vi "Reset_To_Zero.vi"(8 "error in":errorcluster, 11 "X-CAN Session in":refnum<class "X-CAN.lvclass">) -> (0 "error out":errorcluster, 3 "X-CAN Session out":refnum<class "X-CAN.lvclass">)   [LabVIEW 2015]
uses:
  <vilib>/Stratom, Inc/X-CAN for myRIO (API)/X-CAN Class/X-CAN.lvclass
  <vilib>/Stratom, Inc/X-CAN for myRIO (API)/X-CAN Class/Type Definitions/CANFrame.ctl
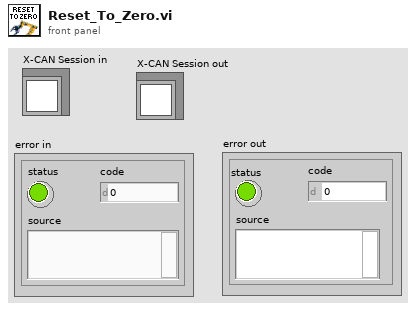
[diagram p1: front panel]
types:
  T1 = typedef "X-CAN.lvclass/CANFrame.ctl" = cluster{"identifier":u32, "extended?":bool, "echo?":bool, "payload":u8[], "timestamp":timestamp}
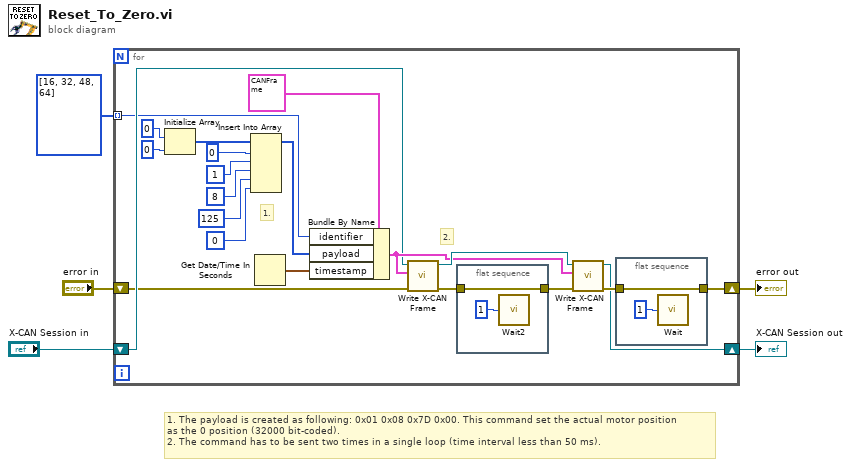
[diagram p0: block diagram]
diagram:
  # "1. The payload is created as following: 0x01 0x08 0x7D 0x00. This command set the actual motor position\nas the 0 position (32000 bit-coded).\n2. The command has to be sent two times in a single loop (time interval less than 50 ms)."
  n1 = for {
    shift-right: [w8] -> w3
    shift-left: "X-CAN Session in" -> [w10]
    shift-right: [w7] -> w2
    shift-left: "error in" -> [w9]
    tunnel: u8[] [16, 32, 48, 64] ("identifier") -> [w6] mode=indexing
    # "2."
    # "1."
    n2 = Initialize Array(u16 0 ("element"), 0 ("dimension size")) -> (w18:u16[])
    n3 = Insert Into Array(array=w18, index=0, new element #1=u8 1 ("new element/subarray"), new element #2=u8 8 ("new element/subarray"), new element #3=u8 125 ("new element/subarray"), new element #4=u8 0 ("new element/subarray")) -> (w15:u16[])
    n4 = Get Date/Time In Seconds() -> (seconds since 1Jan1904=w22:timestamp)
    n5 = Bundle By Name(cluster=T1 {"identifier"=0, "extended?"=FALSE, "echo?"=FALSE, "payload"=[], "timestamp"=timestamp(0 s since 1904-01-01)} ("CAN Frame"), "identifier"=w6, "payload"=w15, "timestamp"=w22) -> (w13:T1)
    n6 = call <vilib>:"Write X-CAN Frame.vi"("error in"=w9, "CAN Frame"=w13, "X-CAN Session in"=w10) -> ("error out"=w24:errorcluster, "X-CAN Session out"=w25:refnum<class "X-CAN.lvclass">)  [unwired: 7 in]
    n7 = flat-sequence {
      tunnel: w24 -> [w27]
      tunnel: [w27] -> w23
      frame #0 {
        n8 = call "Wait2"("Count(mSec)"=u32 1 ("milliseconds to wait")) -> ()  [unwired: 1 out]
      }
    }
    n9 = call <vilib>:"Write X-CAN Frame.vi"("error in"=w23, "CAN Frame"=w13, "X-CAN Session in"=w25) -> ("error out"=w26:errorcluster, "X-CAN Session out"=w8:refnum<class "X-CAN.lvclass">)  [unwired: 7 in]
    n10 = flat-sequence {
      tunnel: w26 -> [w29]
      tunnel: [w29] -> w7
      frame #0 {
        n11 = call "Wait"("Count(mSec)"=u32 1 ("milliseconds to wait")) -> ()  [unwired: 1 out]
      }
    }
  }
  "error out" <- w2
  "X-CAN Session out" <- w3
